vi "3.3.1-Battery Voltage.vi"(11 "Battery Voltage":dbl) -> (3 "3.3.1-Act Command (Battery Voltage)":dbl[](array[numeric]))   [LabVIEW 2010]
uses:
  <vilib>/Analysis/1siggen.llb/Ramp Pattern by Samples.vi
  <vilib>/Analysis/NI_AALBase.lvlib
panel:
  out "Output curve":cluster{dbl[], "Ramp Pattern":dbl[]}(graph)
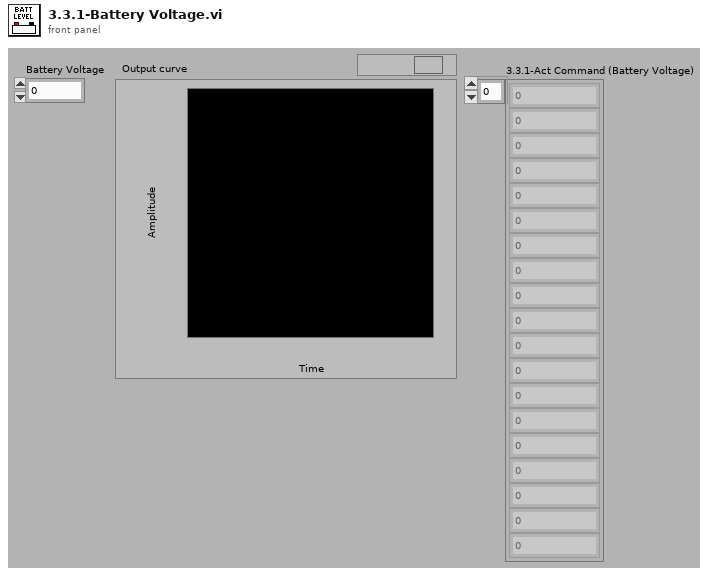
[diagram p1: front panel]
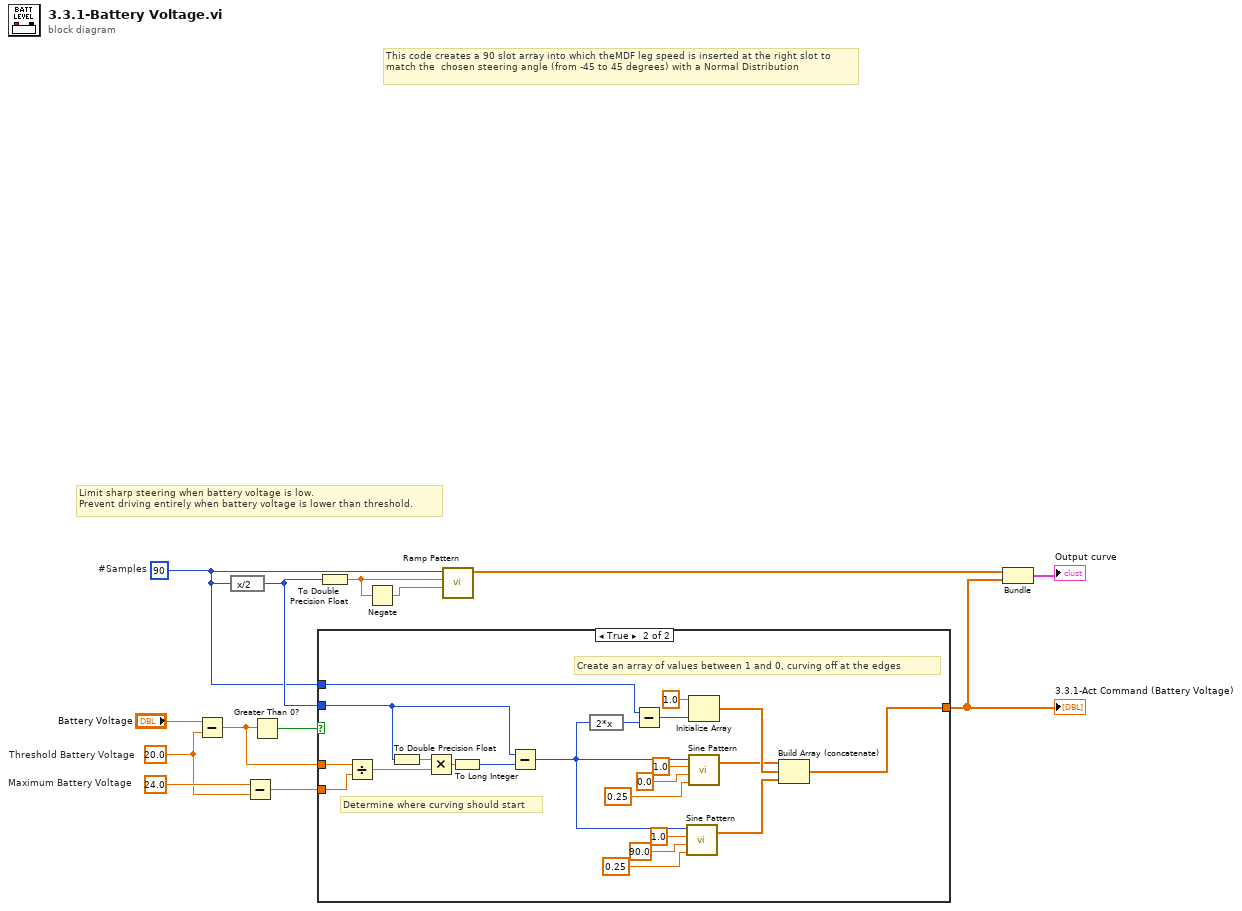
[diagram p0: block diagram]
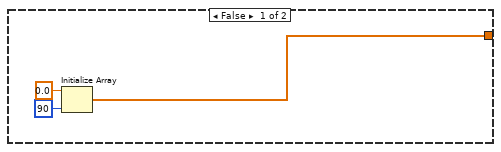
[diagram p2: hidden frame]
diagram:
  w1 = 90  # #Samples
  w5 = 24.0  # Maximum Battery Voltage
  w4 = 20.0  # Threshold Battery Voltage
  # "Limit sharp steering when battery voltage is low.\nPrevent driving entirely when battery voltage is lower than threshold."
  # "This code creates a 90 slot array into which theMDF leg speed is inserted at the right slot to match the  chosen steering angle (from -45 to 45 degrees) with a Normal Distribution"
  n1 = Subtract(x="Battery Voltage", y=w4) -> (x-y=w11:dbl)
  n2 = expression code="x/2"(w1) -> (w2:i32)
  n3 = Subtract(x=w5, y=w4) -> (x-y=w3:dbl)
  n4 = Greater Than 0?(x=w11) -> (x > 0?=w12:bool)
  n5 = case shown="True" w12 {
    tunnel: w11 -> [_ w35]
    tunnel: [w14 w32] -> w8
    tunnel: w3 -> [_ w22]
    tunnel: w2 -> [_ w20]
    tunnel: w1 -> [_ w19]
    frame False {
      n6 = Initialize Array(0.0 ("element"), 90 ("dimension size")) -> (w14:dbl[])
    }
    frame True {
      # "Create an array of values between 1 and 0, curving off at the edges"
      # "Determine where curving should start"
      n7 = Divide(x=w35, y=w22) -> (x/y=w37:dbl)
      n8 = To Double Precision Float(number=w20) -> (double precision float=w21:dbl)
      n9 = Multiply(x=w21, y=w37) -> (x*y=w36:dbl)
      n10 = To Long Integer(number=w36) -> (32bit integer=w38:i32)
      n11 = Subtract(x=w20, y=w38) -> (x-y=w24:i32)
      n12 = expression code="2*x"(w24) -> (w18:i32)
      n13 = Subtract(x=w19, y=w18) -> (x-y=w17:i32)
      n14 = call <vilib>:"Sine Pattern.vi"("cycles"=0.25, "phase(degrees)"=90.0 ("start"), "amplitude"=1.0 ("end"), "samples"=w24) -> ("Sinusoidal Pattern"=w28:dbl[])  [unwired: 1 out]
      n15 = Initialize Array(1.0 ("element"), w17) -> (w33:dbl[])
      n16 = call <vilib>:"Sine Pattern.vi"("cycles"=0.25, "phase(degrees)"=0.0 ("start"), "amplitude"=1.0 ("end"), "samples"=w24) -> ("Sinusoidal Pattern"=w23:dbl[])  [unwired: 1 out]
      n17 = Build Array (concatenate)(w23, w33, w28) -> (w32:dbl[])
    }
  }
  "3.3.1-Act Command (Battery Voltage)" <- w8
  n18 = To Double Precision Float(number=w2) -> (double precision float=w6:dbl)
  n19 = Negate(x=w6) -> (-x=w7:dbl)
  n20 = call-poly <vilib>:"Ramp Pattern.vi"("start"=w7, "end"=w6, "samples"=w1) -> ("Ramp Pattern"=w9:dbl[])  [unwired: 7 in, 1 out]
  n21 = Bundle("Ramp Pattern"=w9, w8) -> (→"Output curve":cluster{"Ramp Pattern":dbl[], dbl[]})  [unwired: 1 in]
